vi "RIMAS Detector Send Configuration.vi"(8 "Error In":errorcluster, 10 "Detector Ref in":refnum<k5>, 11 "Detector Config":T1={"Detector"=0, "Offsets 0"=[0, 0, 0, 0, 0, 0, 0, 0, 0, 0, 0, 0, 0, 0, 0, 0, 0, 0, 0, 0, 0, 0, 0, 0, 0, 0, 0, 0, 0, 0, 0, 0], "Detector Computer"={"Machine"="192.168.121.11", "Password"="", "FITS File Path"="", "Port"=44444, "Header Path"="", "Simulate"=FALSE}, "FITS hdr template0"=path "", "FITS hdr template1"=path "", "FITS Data File Path"=path "", "FITS Detector Settings"={"Exp Time Short"=0.0, "# of Frames"=1.0, "Exp Time Long"=0.0, "# of Groups"=0.0, "Object Name"="", "Object"="", "Obs Type"="", "Image Type"="", "Observer"="", "Observer Affiliation"=""}, "Offsets 1"=[0, 0, 0, 0, 0, 0, 0, 0, 0, 0, 0, 0, 0, 0, 0, 0, 0, 0, 0, 0, 0, 0, 0, 0, 0, 0, 0, 0, 0, 0, 0, 0], "Sim Folder"=path ""} {"Offsets 1" format="%04x"; "Offsets 0" format="%04x"; "Detector" items=["0", "1", "2"]}) -> (0 "Error Out":errorcluster, 1 "log":string, 2 "responses":string[](array[string]), 3 "Detector Ref":refnum<k5>, 5 "Cmds executed":string[](array[string]))   [LabVIEW 2020]
uses:
  RIMAS Detector Config.ctl
  RIMAS Detector Server Config.ctl
  RIMAS Observation Config.ctl
panel:
  out "Status Controllers":string
  out "Status Headers":string
  out "Array":i32[](array[numeric])
  # "sec"
  # "sec"
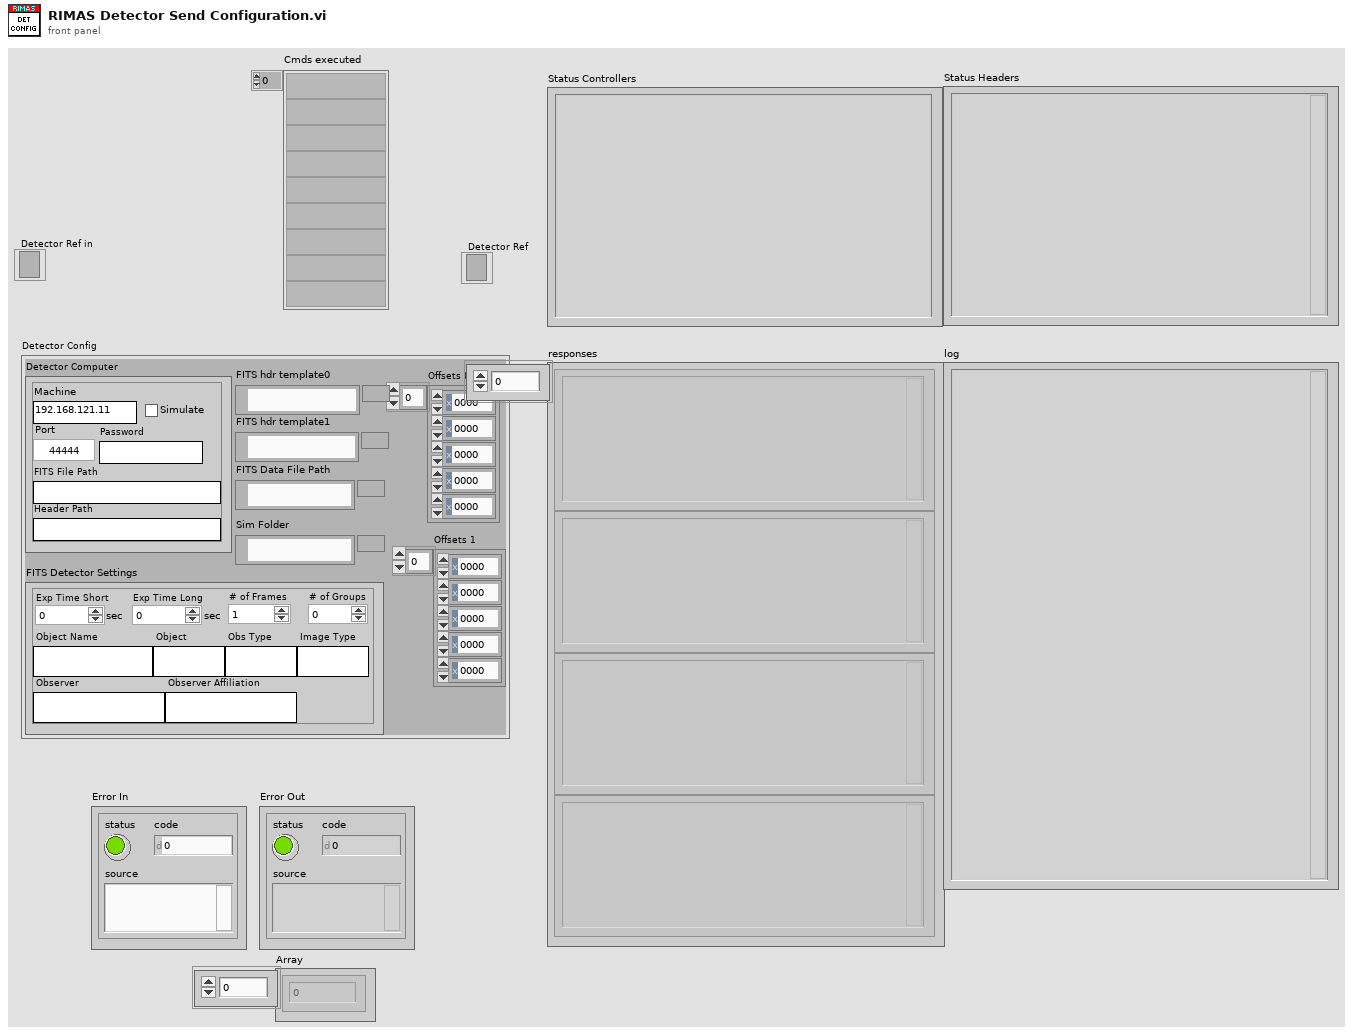
[diagram p1: front panel]
types:
  T1 = typedef "RIMAS Detector Config.ctl" = cluster{"Detector":u16, "Offsets 0":u16[], "Detector Computer":T2, "FITS hdr template0":path, "FITS hdr template1":path, "FITS Data File Path":path, "FITS Detector Settings":T3, "Offsets 1":u16[], "Sim Folder":path}
  T2 = typedef "RIMAS Detector Server Config.ctl" = cluster{"Machine":string, "Password":string, "FITS File Path":string, "Port":u16, "Header Path":string, "Simulate":bool}
  T3 = typedef "RIMAS Observation Config.ctl" = cluster{"Exp Time Short":dbl, "# of Frames":dbl, "Exp Time Long":dbl, "# of Groups":dbl, "Object Name":string, "Object":string, "Obs Type":string, "Image Type":string, "Observer":string, "Observer Affiliation":string}
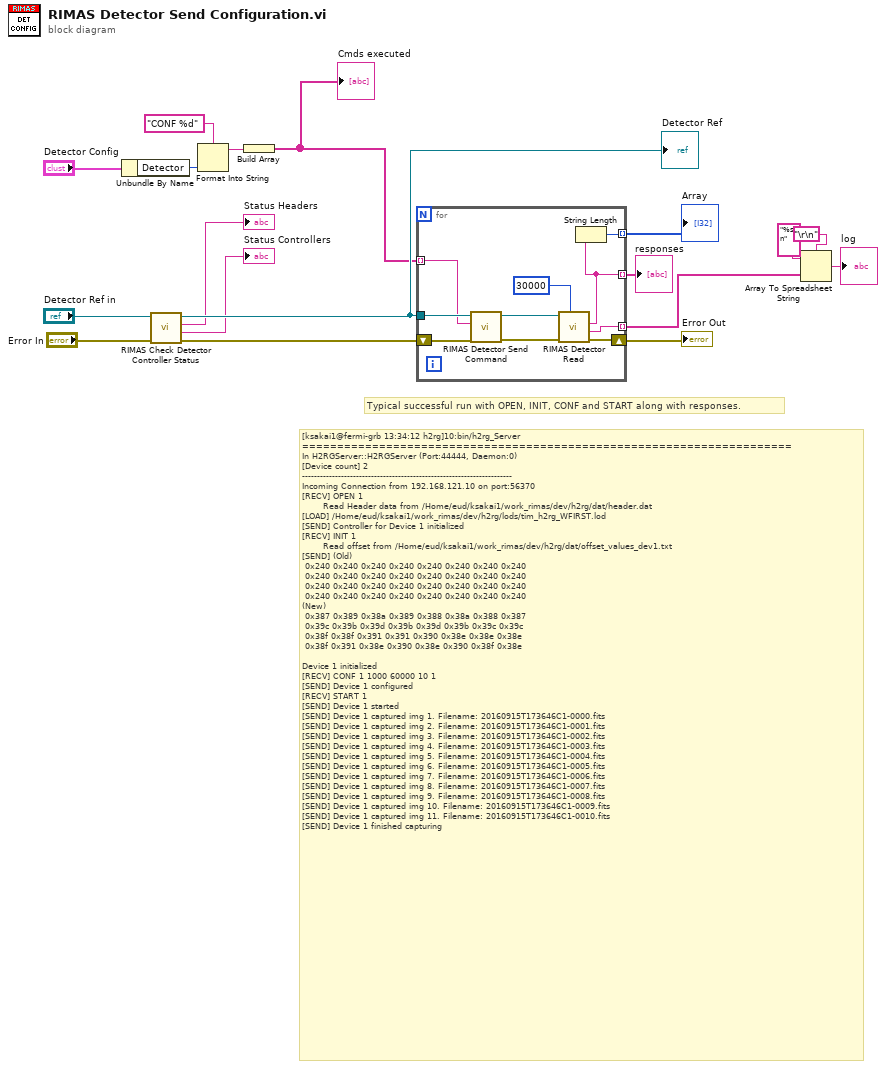
[diagram p0: block diagram]
diagram:
  # "Typical successful run with OPEN, INIT, CONF and START along with responses."
  # "[ksakai1@fermi-grb 13:34:12 h2rg]10:bin/h2rg_Server\n======================================================================\nIn H2RGServer::H2RGServer (Port:44444, Daemon:0)\n[Device count] 2\n----------------------------------------------------------------------\nIncoming Connection from 192.168.121.10 on port:56370\n[RECV] OPEN 1\n       Read Header data from /Home/eud/ksakai1/work_rimas/dev/h2rg/dat/header.dat\n[LOAD] /Home/eud/ksakai1/work_rimas/dev/h2rg/lods/tim_h2rg_WFIRST.lod\n[SEND] Controller for Device 1 initialized\n[RECV] INIT 1\n       Read offset from /Home/eud/ksakai1/work_rimas/dev/h2rg/dat/offset_values_dev1.txt\n[SEND] (Old)\n 0x240 0x240 0x240 0x240 0x240 0x240 0x240 0x240\n 0x240 0x240 0x240 0x240 0x240 0x240 0x240 0x240\n 0x240 0x240 0x240 0x240 0x240 0x240 0x240 0x240\n 0x240 0x240 0x240 0x240 0x240 0x240 0x240 0x240\n(New)\n 0x387 0x389 0x38a 0x389 0x388 0x38a 0x388 0x387\n 0x39c 0x39b 0x39d 0x39b 0x39d 0x39b 0x39c 0x39c\n 0x38f 0x38f 0x391 0x391 0x390 0x38e 0x38e 0x38e\n 0x38f 0x391 0x38e 0x390 0x38e 0x390 0x38f 0x38e\n\nDevice 1 initialized\n[RECV] CONF 1 1000 60000 10 1\n[SEND] Device 1 configured\n[RECV] START 1\n[SEND] Device 1 started\n[SEND] Device 1 captured img 1. Filename: 20160915T173646C1-0000.fits\n[SEND] Device 1 captured img 2. Filename: 20160915T173646C1-0001.fits\n[SEND] Device 1 captured img 3. Filename: 20160915T173646C1-0002.fits\n[SEND] Device 1 captured img 4. Filename: 20160915T173646C1-0003.fits\n[SEND] Device 1 captured img 5. Filename: 20160915T173646C1-0004.fits\n[SEND] Device 1 captured img 6. Filename: 20160915T173646C1-0005.fits\n[SEND] Device 1 captured img 7. Filename: 20160915T173646C1-0006.fits\n[SEND] Device 1 captured img 8. Filename: 20160915T173646C1-0007.fits\n[SEND] Device 1 captured img 9. Filename: 20160915T173646C1-0008.fits\n[SEND] Device 1 captured img 10. Filename: 20160915T173646C1-0009.fits\n[SEND] Device 1 captured img 11. Filename: 20160915T173646C1-0010.fits\n[SEND] Device 1 finished capturing"
  n1 = Unbundle By Name("Detector Config") -> ("Detector"=w15:u16)
  n2 = call "RIMAS Check Detector Controller Status.vi"("error in (no error)"="Error In", "Detector Ref  in"="Detector Ref in") -> ("error out"=w7:errorcluster, "Status Controllers"=→"Status Controllers":string, "Status Headers"=→"Status Headers":string, "Detector Ref out"=w5:refnum<k5>)  [unwired: 6 in]
  "Detector Ref" <- w5
  n3 = Format Into String(format string="CONF %d", w15) -> (resulting string=w2:string)  [unwired: 2 in, 1 out]
  n4 = Build Array(w2) -> (w1:string[])
  "Cmds executed" <- w1
  n5 = for {
    shift-right: [w23] -> w18
    shift-left: w7 -> [w28]
    tunnel: w5 -> [w27]
    tunnel: w1 -> [w26] mode=indexing
    tunnel: [w22] -> w11 mode=indexing
    tunnel: [w21] -> w14 mode=indexing
    tunnel: [w19] -> w9 mode=indexing
    n6 = call "RIMAS Detector Send Command.vi"("Error In"=w28, "Command"=w26, "Detector Ref"=w27) -> ("Error Out"=w25:errorcluster, "Detector Ref dup"=w24:refnum<k5>)  [unwired: 6 in, 1 out]
    n7 = call "RIMAS Detector Read.vi"("timeout (ms)"=30000, "Error In"=w25, "Detector Ref"=w24) -> ("Error Out"=w23:errorcluster, "First String"=w19:string, "data out"=w22:string)  [unwired: 5 in, 1 out]
    n8 = String Length(string=w22) -> (length=w21:i32)
  }
  "Error Out" <- w18
  "responses" <- w11
  "Array" <- w14
  n9 = Array To Spreadsheet String(delimiter (Tab)="\r\n", array=w9, 3:"%s\n" ("format string")) -> (spreadsheet string=→"log":string)
